vi "EnumerateMethods.vi"(8 "error in (no error)":errorcluster) -> (0 "error out":errorcluster, 1 "Method Helps":string[](array[string]), 2 "Service Name":string, 3 "Methods":string[](array[string]))   [LabVIEW 2020, in "WebServiceImporter.lvlib" / "ProxyDll Generator.lvlib"]
doc: "Get the name of the Web Service and array of method names"
uses:
  <vilib>/Platform/WebService/ProxyDll Generator/ProxyDll Generator.lvlib
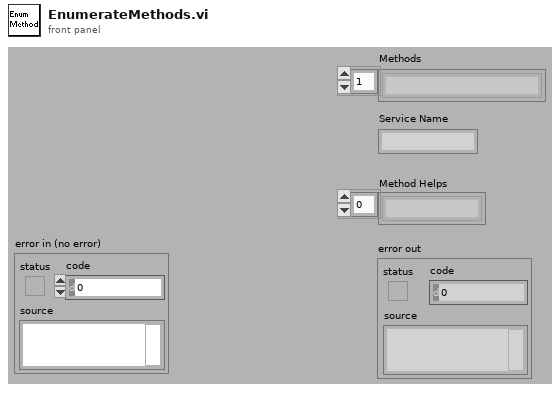
[diagram p1: front panel]
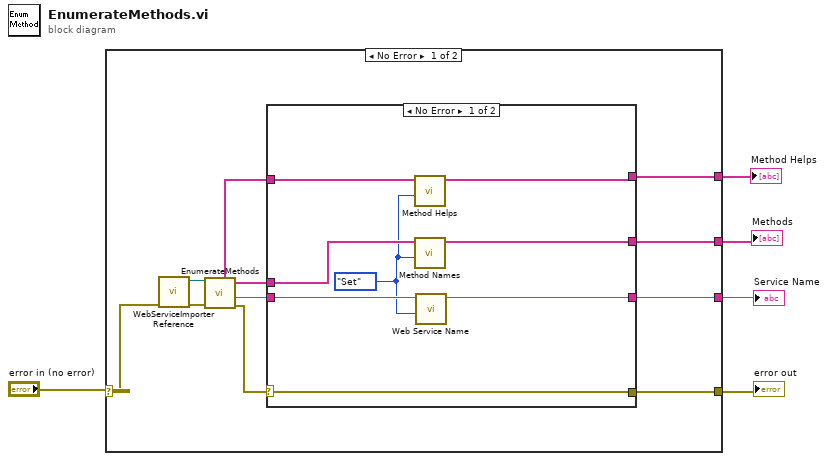
[diagram p0: block diagram]
diagram:
  n1 = case shown="No Error" "error in (no error)" {
    selector: "error in (no error)" -> [w8 w26]
    tunnel: [w13 w26] -> w4
    tunnel: [w11 _] -> w3
    tunnel: [w10 _] -> w2
    tunnel: [w6 _] -> w1
    frame No Error {
      n2 = call <vilib>:"WebServiceImporter Reference.vi"("error in (no error)"=w8) -> ("error out"=w9:errorcluster, "Web Service Importer out"=w16:refnum<k24>)  [unwired: 9 in]
      n3 = call <vilib>:"EnumerateMethods.vi"("error in (no error)"=w9, "Web Service Importer in"=w16) -> ("error out"=w15:errorcluster, "ServiceName"=w12:string, "Methods"=w14:string[], "MethodsHelp"=w7:string[])  [unwired: 5 in, 1 out]
      n4 = case shown="No Error" w15 {
        selector: w15 -> [w20 w25]
        tunnel: w14 -> [w24 _]
        tunnel: [w20 w25] -> w13
        tunnel: w12 -> [w23 _]
        tunnel: [w22 _] -> w11
        tunnel: [w21 _] -> w10
        tunnel: w7 -> [w19 _]
        tunnel: [w17 _] -> w6
        frame No Error {
          w18 = enum16{"Get", "Set"}."Set" ("Operation")
          n5 = call <vilib>:"Method Helps.vi"("Operation"=w18, "Method Helps"=w19) -> ("Method Helps (out)"=w17:string[])  [unwired: 8 in, 1 out]
          n6 = call <vilib>:"Method Names.vi"("Operation"=w18, "Method Names"=w24) -> ("Method Names (out)"=w22:string[])  [unwired: 8 in, 1 out]
          n7 = call <vilib>:"Web Service Name.vi"("Operation"=w18, "Web Service Name"=w23) -> ("Web Service Name (out)"=w21:string)  [unwired: 8 in, 1 out]
        }
        frame Error {
        }
      }
    }
    frame Error {
    }
  }
  "error out" <- w4
  "Methods" <- w3
  "Service Name" <- w2
  "Method Helps" <- w1
